vi "Insert Event.vi"(0 "Event queue in":string[](array[string]), 1 "Replace all？（F）":bool, 2 "Insert Selected?":bool[](array[boolean]), 3 "Insert all? (T)":bool=TRUE, 4 "Events to Insert":string[](array[string])) -> (7 "Event queue out":string[](array[string]))   [LabVIEW 2018]
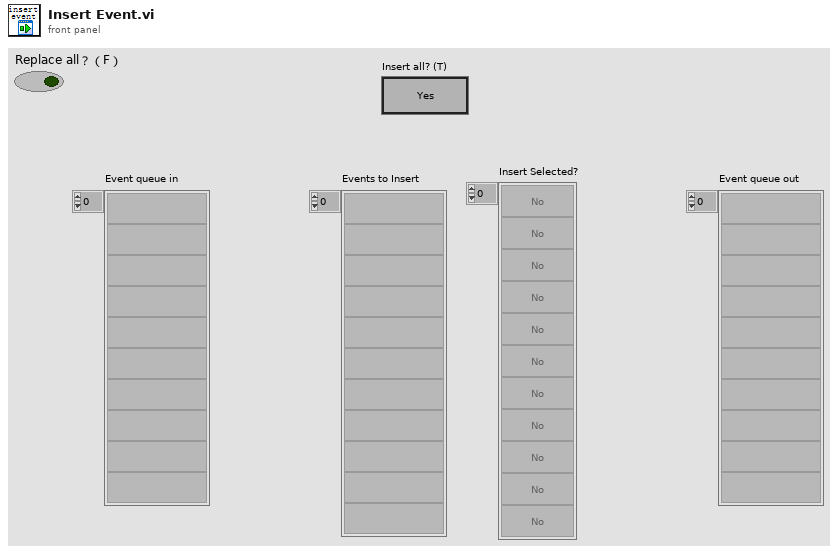
[diagram p1: front panel]
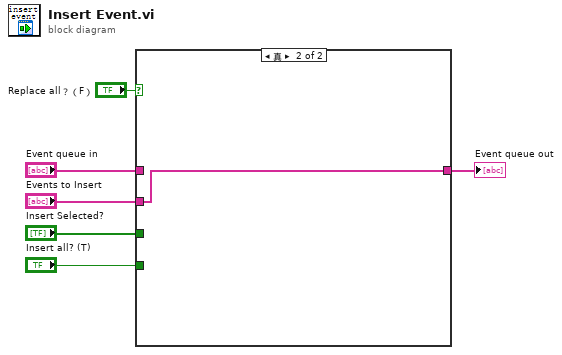
[diagram p0: block diagram]
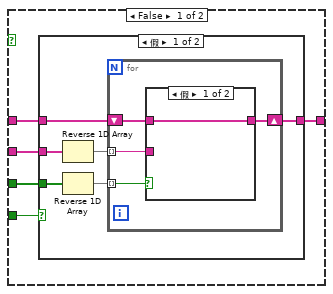
[diagram p2: hidden frame]
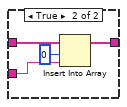
[diagram p3: hidden frame]
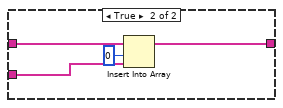
[diagram p4: hidden frame]
diagram:
  n1 = case shown="真" "Replace all？（F）" {
    tunnel: "Event queue in" -> [w11 _]
    tunnel: [w10 w31] -> w5
    tunnel: "Insert all? (T)" -> [w9 _]
    tunnel: "Events to Insert" -> [w8 w31]
    tunnel: "Insert Selected?" -> [w7 _]
    frame False {
      n2 = case shown="假" w9 {
        tunnel: w11 -> [w17 w30]
        tunnel: [w16 w27] -> w10
        tunnel: w7 -> [w13 _]
        tunnel: w8 -> [w15 w28]
        frame False {
          n3 = Reverse 1D Array(array=w15) -> (reversed array=w14:string[])
          n4 = Reverse 1D Array(array=w13) -> (reversed array=w12:bool[])
          n5 = for {
            tunnel: w14 -> [w21] mode=indexing
            tunnel: w12 -> [w18] mode=indexing
            shift-right: [w19] -> w16
            shift-left: w17 -> [w20]
            n6 = case shown="假" w18 {
              tunnel: w21 -> [_ w25]
              tunnel: [w22 w24] -> w19
              tunnel: w20 -> [w22 w26]
              frame False {
              }
              frame True {
                n7 = Insert Into Array(array=w26, index=0 ("Index"), new element=w25) -> (w24:string[])
              }
            }
          }
        }
        frame True {
          n8 = Insert Into Array(array=w30, index=0 ("Index"), new element=w28) -> (w27:string[])
        }
      }
    }
    frame True {
    }
  }
  "Event queue out" <- w5
